vi "subMoveDetect.vi"(0 "X":dbl format="%#_13g", 1 "Upper\nTolerance":dbl=1.0 format="%#.13g", 2 "Y":dbl format="%#_13g", 3 "Z":dbl format="%#_13g", 4 "Lower\nTolerance":dbl=1.0 format="%#.3g") -> (5 "Movement Event Array":bool[](array[boolean]))   [LabVIEW 2017]
doc: "The subMoveDetect programme is a subVI which usues the myRIO onboard accelerometer to detect movement of the unit and allows control of the sensitivity limits to enable boolean flags to be set if the movement threshold exceeds these limits."
panel:
  # "This VI collects information from three inputs and looks\nfor changes between ranges, as set by the tolerances.\nIt outputs true/false to an array."
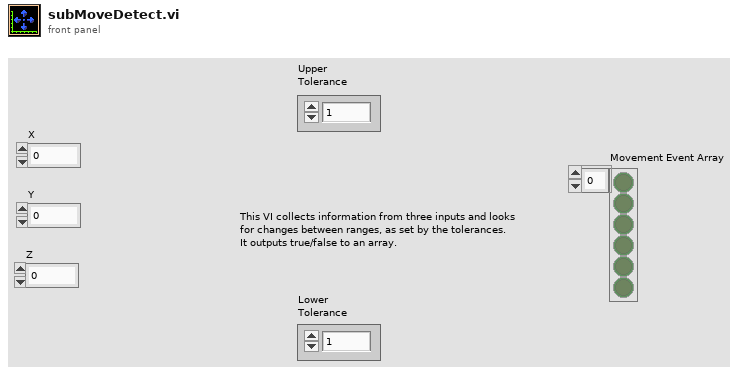
[diagram p1: front panel]
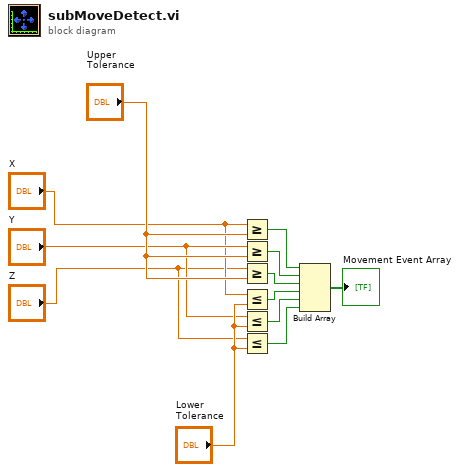
[diagram p0: block diagram]
diagram:
  n1 = Greater Or Equal?(x="X", y="Upper\nTolerance") -> (x >= y?=w12:bool)
  n2 = Greater Or Equal?(x="Y", y="Upper\nTolerance") -> (x >= y?=w11:bool)
  n3 = Greater Or Equal?(x="Z", y="Upper\nTolerance") -> (x >= y?=w10:bool)
  n4 = Less Or Equal?(x="X", y="Lower\nTolerance") -> (x <= y?=w9:bool)
  n5 = Less Or Equal?(x="Y", y="Lower\nTolerance") -> (x <= y?=w8:bool)
  n6 = Less Or Equal?(x="Z", y="Lower\nTolerance") -> (x <= y?=w7:bool)
  n7 = Build Array(w12, w11, w10, w9, w8, w7) -> (→"Movement Event Array":bool[])
